vi "sv_Preprocess Shock Signal.vi"(8 "error in (no error)":errorcluster, 10 "preprocessing settings":T1 {"lowpass cutoff frequency [Hz]" format="%.2f"}, 11 "scaled signal [EU]":waveform(dbl)) -> (0 "error out":errorcluster, 3 "filtered scaled signal [EU]":waveform(dbl))   [LabVIEW 2017, in "SoundVib_Transient.lvlib"]
doc: "Preprocesses <B>signal in</B> by performing lowpass filtering and removing the DC offset."
uses:
  <vilib>/addons/Sound and Vibration/svt_Transients/SoundVib_Transient.lvlib
  <vilib>/Analysis/baseanly.llb/Mean (DBL).vi
  <vilib>/Waveform/WDTOps.llb/WDT Get Waveform Subset DBL (LV80).vi
  <vilib>/Waveform/WDTOps.llb/WDT Number of Waveform Samples DBL.vi
  <vilib>/measure/macond.llb/FIR Filter for 1 Chan.vi
  <vilib>/measure/NI_MAPro.lvlib
  <vilib>/Analysis/NI_AALBase.lvlib
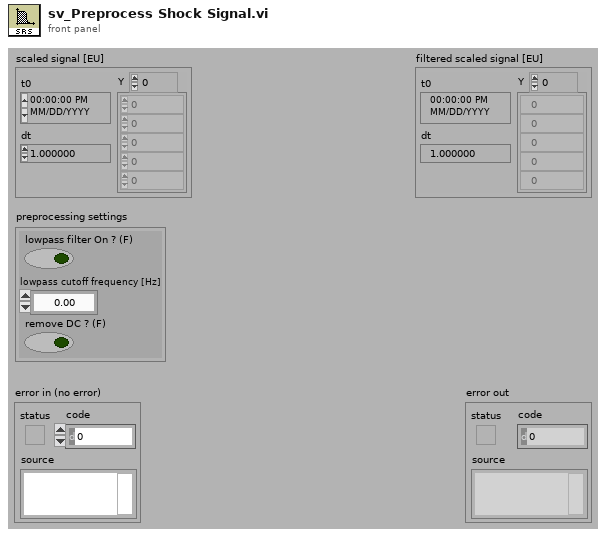
[diagram p1: front panel]
types:
  T1 = cluster{"lowpass filter On ? (F)":bool, "lowpass cutoff frequency [Hz]":dbl, "remove DC ? (F)":bool}
  T2 = cluster{"Topology":enum16{"Off", "FIR by Specification", "Equi-ripple FIR", "Windowed FIR"}, "Type":enum16{"Lowpass", "Highpass", "Bandpass", "Bandstop"}, "#Taps":i32, "Lower PB":dbl, "Upper PB":dbl, "Lower SB":dbl, "Upper SB":dbl}
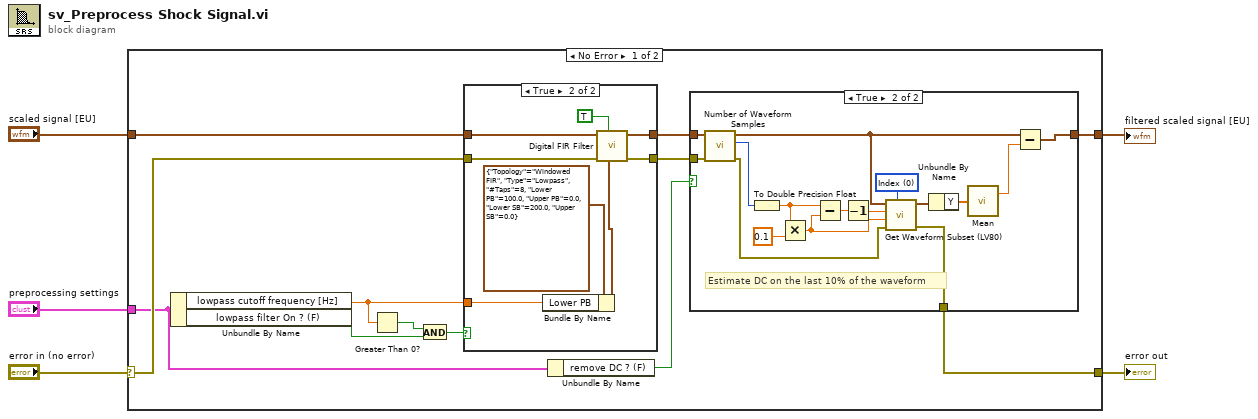
[diagram p0: block diagram]
diagram:
  n1 = case shown="No Error" "error in (no error)" {
    selector: "error in (no error)" -> [w16 w47]
    tunnel: [w14 w47] -> w4
    tunnel: "scaled signal [EU]" -> [w13 w46]
    tunnel: "preprocessing settings" -> [w8 _]
    tunnel: [w6 w46] -> w1
    frame No Error {
      n2 = Unbundle By Name(w8) -> ("lowpass cutoff frequency [Hz]"=w12:dbl, "lowpass filter On ? (F)"=w10:bool)
      n3 = Greater Than 0?(x=w12) -> (x > 0?=w11:bool)
      n4 = And(x=w11, y=w10) -> (x .and. y?=w9:bool)
      n5 = case shown="True" w9 {
        tunnel: [w37 w45] -> w17
        tunnel: w12 -> [_ w38]
        tunnel: w13 -> [w37 w39]
        tunnel: w16 -> [w36 w41]
        tunnel: [w36 w40] -> w15
        frame False {
        }
        frame True {
          n6 = Bundle By Name(cluster=T2 {"Topology"=enum."Windowed FIR", "Type"=enum."Lowpass", "#Taps"=8, "Lower PB"=100.0, "Upper PB"=0.0, "Lower SB"=200.0, "Upper SB"=0.0} ("FIR filter specifications"), "Lower PB"=w38) -> (w43:T2)
          n7 = call-poly <vilib>:"Digital FIR Filter.vi"("FIR filter specifications"=w43, "reset filter"=TRUE, "error in (no error)"=w41, "signal in"=w39) -> ("error out"=w40:errorcluster, "signal out"=w45:waveform(dbl))  [unwired: 5 in, 1 out]
        }
      }
      n8 = Unbundle By Name(w8) -> ("remove DC ? (F)"=w7:bool)
      n9 = case shown="True" w7 {
        tunnel: w17 -> [w19 w35]
        tunnel: [w19 w30] -> w6
        tunnel: w15 -> [w18 w29]
        tunnel: [w18 w20] -> w14
        frame False {
        }
        frame True {
          w24 = u16 0 items=["Index", "Relative Time"] ("Mode")
          # "Estimate DC on the last 10% of the waveform"
          n10 = call-poly <vilib>:"Number of Waveform Samples.vi"("error in (no error)"=w29, "waveform in"=w35) -> ("error out"=w21:errorcluster, "number of samples"=w33:i32, "waveform out"=w25:waveform(dbl))  [unwired: 7 in]
          n11 = To Double Precision Float(number=w33) -> (double precision float=w28:dbl)
          n12 = Multiply(x=w28, y=0.1) -> (x*y=w22:dbl)
          n13 = Subtract(x=w28, y=w22) -> (x-y=w32:dbl)
          n14 = Decrement(x=w32) -> (x-1=w23:dbl)
          n15 = call-poly <vilib>:"Get Waveform Subset (LV80).vi"("start/duration format"=w24, "error in (no error)"=w21, "duration"=w22, "start samples/time"=w23, "waveform in"=w25) -> ("error out"=w20:errorcluster, "waveform out"=w26:waveform(dbl))  [unwired: 1 in, 2 out]
          n16 = Unbundle By Name(w26) -> ("Y"=w31:dbl[])
          n17 = call-poly <vilib>:"Mean.vi"("X"=w31) -> ("mean"=w27:dbl)  [unwired: 1 out]
          n18 = Subtract(x=w25, y=w27) -> (x-y=w30:waveform(dbl))
        }
      }
    }
    frame Error {
    }
  }
  "error out" <- w4
  "filtered scaled signal [EU]" <- w1
